vi "soma_com_subvi.vi"() -> ()   [LabVIEW 2018]
panel:
  out "(x+10)*y":dbl
  out "x+10":dbl
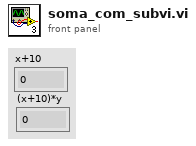
[diagram p1: front panel]
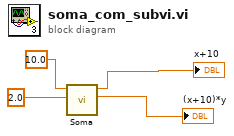
[diagram p0: block diagram]
diagram:
  n1 = call "Soma.vi"("y"=2.0, "x"=10.0) -> ("(x+10)*y"=→"(x+10)*y":dbl, "x+10"=→"x+10":dbl)  [unwired: 8 in]
